vi "devide_by_0_indicator.vi"() -> ()   [LabVIEW 2015]
panel:
  out "Boolean":bool
  out "output":dbl
  in  "no.2":dbl
  in  "no.1":dbl
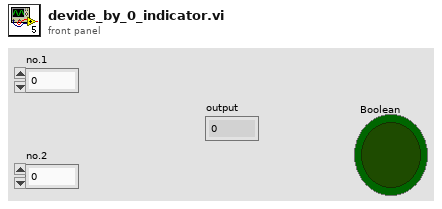
[diagram p1: front panel]
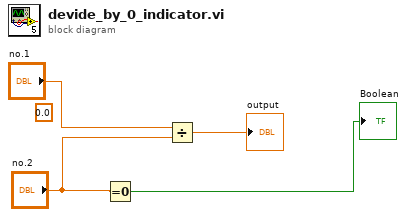
[diagram p0: block diagram]
diagram:
  (unwired) 0.0 ("Numeric")
  n1 = Equal To 0?(x="no.2") -> (x = 0?=→"Boolean":bool)
  n2 = Divide(x="no.1", y="no.2") -> (x/y=→"output":dbl)
